vi "Tosca-DI Acq Thread.vi"(0 "Input Events":T2[](array[typedef]), 1 "Action":enum16{"Stop", "Preview", "Run"}(ring), 7 "Digital Inputs in":T1[](array[typedef]), 11 "Acq Data":refnum<queue>) -> (15 "error out":errorcluster)   [LabVIEW 2020]
uses:
  Tosca-Input Event.ctl
  Tosca-Input Criterion.ctl
  epl-vi-lib/Utility VIs/Type Defs/Logic State.ctl
  Typedefs/Tosca-Accumulator.ctl
  Tosca-Digital Input.ctl
  Tosca-DI Acq Data.ctl
  <vilib>/Platform/TimedLoop/XDataNode/timing_clust.ctl
  <vilib>/Platform/TimedLoop/XDataNode/nitl_modes.ctl
  <vilib>/Platform/TimedLoop/XDataNode/wakeup.ctl
  <vilib>/DAQmx/read.llb/DAQmx Read.vi
  <vilib>/DAQmx/read.llb/DAQmx Read (Digital 1D Bool NChan 1Samp 1Line).vi
  Tosca-Evaluate Criterion.vi
  Sub VIs/Tosca-Process Event Accumulation.vi
  Sub VIs/Tosca-Process Event Accumulation.vi/57260889-9eb4-4fe2-974f-94be7248788a.vi
  Sub VIs/Tosca-Globals.vi
  <vilib>/DAQmx/miscellaneous.llb/DAQmx Fill In Error Info.vi
  <vilib>/Platform/TimedLoop/XDataNode/XDataNode.xnode
  <vilib>/Platform/TimedLoop/XDataNode/XDNodeRunTimeDep.lvlib
panel:
  in  "error in (no error)":errorcluster
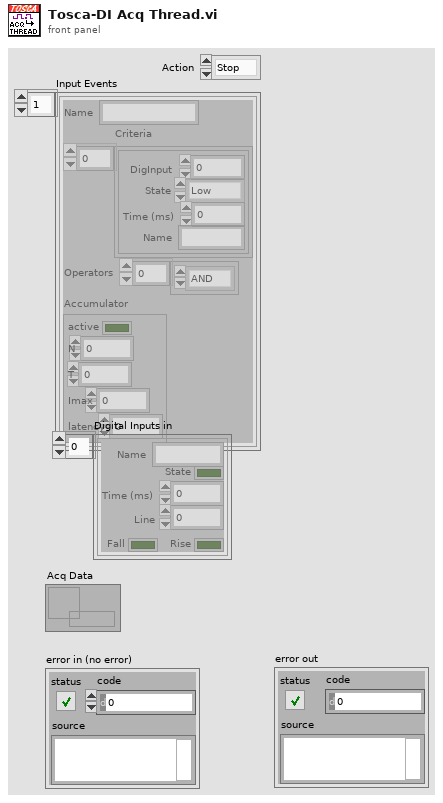
[diagram p1: front panel]
types:
  T1 = typedef "Tosca-Digital Input.ctl" = cluster{"Name":string, "State":bool, "Time (ms)":dbl, "Line":i32, "Rise":bool, "Fall":bool}
  T2 = typedef "Tosca-Input Event.ctl" = cluster{"Name":string, "Criteria":T3[], "Operators":enum16{"AND", "OR"}[], "Accumulator":T5}
  T3 = typedef "Tosca-Input Criterion.ctl" = cluster{"DigInput":i32, "State":T4, "Time (ms)":i32, "Name":string}
  T4 = typedef "Logic State.ctl" = enum16{"Low", "High", "Rising", "Falling"}
  T5 = typedef "Tosca-Accumulator.ctl" = cluster{"active":bool, "N":i32, "T":dbl, "Imax":dbl, "latency":dbl}
  T6 = typedef "XDNodeRunTimeDep.lvlib/timing_clust.ctl" = cluster{"Expected End [f-1]":u64, "Actual End [f-1]":u64, "Finished Late? [f-1]":bool, "Expected End [i-1]":u64, "Actual End [i-1]":u64, "Finished Late? [i-1]":bool, "Expected Start [i]":u64, "Actual Start [i]":u64, "Expected Start [f]":u64, "Actual Start [f]":u64, "Source Name":string, "Structure Name":string, "Period":i64, "Deadline":i64, "Offset":i64, "Start":i64, "Priority":i32, "Timeout":i32, "Mode":T7, "Wakeup Reason":T8, "Error":errorcluster, "Source Type":string, "Secondary Source Type":string, "Global End Time":u64, "Global Start Time":u64, "Frame Duration":u64, "Iteration Duration":u64, "Assigned CPU":i32, "I/O Scan Engine Mode":u32}
  T7 = typedef "XDNodeRunTimeDep.lvlib/nitl_modes.ctl" = enum32{"No Change", "Process missed periods, maintain original phase", "Discard missed periods, maintain original phase", "Process missed periods, ignore original phase", "Discard missed periods, ignore original phase"}
  T8 = typedef "XDNodeRunTimeDep.lvlib/wakeup.ctl" = enum32{"Normal", "Aborted", "Asynchronous wakeup", "Timing source error", "Timed loop error", "Timeout"}
  T9 = typedef "Tosca-Accumulator State.ctl" = cluster{"last":bool, "times":dbl[], "tstate":dbl}
  T10 = cluster{"Period":i64, dbl, "DI out":bool[], "Events":bool[], dbl, bool}
  T11 = typedef "Tosca-DI Acq Data.ctl" = cluster{"dt":i64, "loop":dbl, "digital":bool[], "events":bool[], "time":dbl, "overtime":bool}
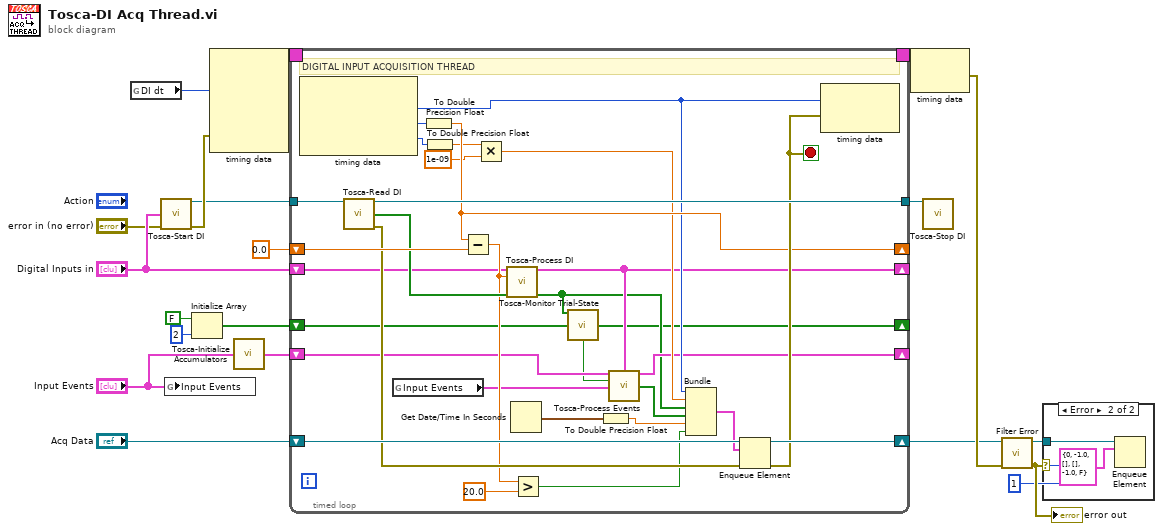
[diagram p0: block diagram]
diagram:
  n1 = global read "Tosca-Globals.vi" "DI dt"() -> (w6:i32)
  n2 = call "Tosca-Start DI.vi"("Digital Inputs"="Digital Inputs in", "error in"="error in (no error)") -> ("Task"=w7:refnum<k21>, "error out"=w14:errorcluster)  [unwired: 12 in]
  n3 = global write "Tosca-Globals.vi" "Input Events"("Input Events") -> ()
  n4 = Initialize Array(FALSE, 2 ("dimension size")) -> (w2:bool[])
  n5 = node-c288(w6, w14) -> (w19:T6)  [unwired: 3 in]
  n6 = call "Tosca-Initialize Accumulators.vi"("Input Events"="Input Events") -> ("Accumulators"=w5:T9[])  [unwired: 14 in]
  n7 = timed-loop {
    timing: w19 -> [_]
    timing-out: [_] -> w18
    shift-right: [w27] -> _
    shift-left: "Digital Inputs in" -> [w28]
    shift-right: [w41] -> _
    shift-left: 0.0 -> [w47]
    tunnel: w7 -> [w50]
    tunnel: [w49] -> w8
    shift-right: [w44] -> w12
    shift-left: "Acq Data" -> [w45]
    shift-right: [w25] -> _
    shift-left: w5 -> [w26]
    shift-right: [w21] -> _
    shift-left: w2 -> [w22]
    stop <- w42 stop-if-true
    # "DIGITAL INPUT ACQUISITION THREAD"
    n8 = node-c288() -> (w37:i64, w48:i64, w40:i64)  [unwired: 1 in, 1 out]
    n9 = call "Tosca-Read DI.vi"("Task in"=w50) -> ("Task out"=w49:refnum<k21>, "data"=w46:bool[], "error out"=w43:errorcluster)  [unwired: 12 in]
    n10 = global read "Tosca-Globals.vi" "Input Events"() -> (w20:T2[])
    n11 = To Double Precision Float(number=w48) -> (double precision float=w41:dbl)
    n12 = To Double Precision Float(number=w40) -> (double precision float=w39:dbl)
    n13 = Subtract(x=w41, y=w47) -> (x-y=w31:dbl)
    n14 = Multiply(x=w39, y=1e-09) -> (x*y=w36:dbl)
    n15 = call "Tosca-Process DI.vi"("Digital Inputs in"=w28, "Interval (ms)"=w31, "DI"=w46) -> ("Digital Inputs out"=w27:T1[], "DI out"=w24:bool[])  [unwired: 11 in]
    n16 = Get Date/Time In Seconds() -> (seconds since 1Jan1904=w33:timestamp)
    n17 = Greater?(x=w31, y=20.0) -> (0:w29:bool)
    n18 = call "Tosca-Monitor Trial-State.vi"("DI"=w24, "Trial/State In"=w22) -> ("Trial/State out"=w21:bool[], "State change?"=w23:bool)  [unwired: 11 in, 1 out]
    n19 = To Double Precision Float(number=w33) -> (double precision float=w32:dbl)
    n20 = call "Tosca-Process Events.vi"("Accum States in"=w26, "Digital Inputs"=w27, "state change"=w23, "Input Events"=w20) -> ("Accum States out"=w25:T9[], "Events"=w35:bool[])  [unwired: 10 in]
    n21 = Bundle("Period"=w37, w36, "DI out"=w24, "Events"=w35, w32, w29) -> (w34:T10)  [unwired: 1 in]
    n22 = Enqueue Element(queue=w45, element=w34, error in (no error)=w43) -> (queue out=w44:refnum<queue>, error out=w42:errorcluster)  [unwired: 1 in, 1 out]
    n23 = node-c288(w37, w42) -> ()  [unwired: 1 out]
  }
  n24 = node-c288(w18) -> (w15:errorcluster)
  n25 = call "Tosca-Stop DI.vi"("Refnum in"=w8) -> ()  [unwired: 15 in]
  n26 = call "Filter Error.vi"("error in (no error)"=w15, "code to ignore"=1) -> ("error out"=w16:errorcluster)  [unwired: 9 in]
  "error out" <- w16
  n27 = case shown="Error" w16 {
    tunnel: w12 -> [_ w60]
    frame No Error {
    }
    frame Error {
      n28 = Enqueue Element(queue=w60, element=T11 {"dt"=0, "loop"=-1.0, "digital"=[], "events"=[], "time"=-1.0, "overtime"=FALSE}) -> ()  [unwired: 2 in, 3 out]
    }
  }
